vi "Read Analog Input Values.vi"(8 "error in":errorcluster, 9 "Timeout / s":dbl=10.0 format="%0.2f", 10 "AI DAQmx Task":refnum<k21>, 11 "BNT_DAQmx-MCSV in":refnum<class "BNT_DAQmx-MCSV.lvclass">) -> (0 "error out":errorcluster, 1 "AI Data":dbl[](array[numeric]), 3 "BNT_DAQmx-MCSV out":refnum<class "BNT_DAQmx-MCSV.lvclass">)   [LabVIEW 2017, in "BNT_DAQmx.lvlib" / "BNT_DAQmx-MCSV.lvclass"]
doc: "Read analog input.\n\n<b>Default Implementation:</b> Analog Input\n\nThis dynamic dispatch VI can be overritten by derived classes to implement other analog input readings."
uses:
  BNT_DAQmx-MCSV.lvclass
  <vilib>/DAQmx/read.llb/DAQmx Read (Analog 1D DBL NChan 1Samp).vi
  <vilib>/DAQmx/miscellaneous.llb/DAQmx Fill In Error Info.vi
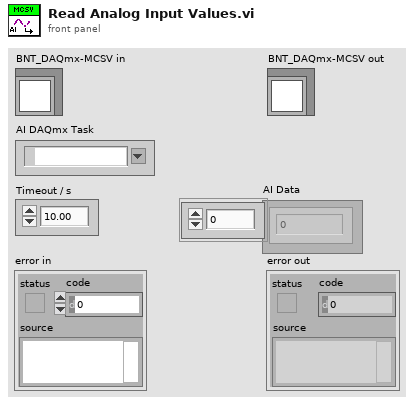
[diagram p1: front panel]
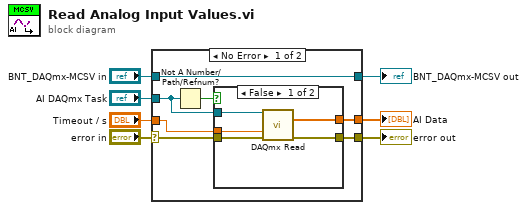
[diagram p0: block diagram]
diagram:
  n1 = case shown="No Error" "error in" {
    selector: "error in" -> [w13 w22]
    tunnel: [w12 w22] -> w6
    tunnel: [w10 w21] -> w4
    tunnel: "BNT_DAQmx-MCSV in" -> [w10 w21]
    tunnel: "Timeout / s" -> [w14 _]
    tunnel: [w11 _] -> w2
    tunnel: "AI DAQmx Task" -> [w8 _]
    frame No Error {
      n2 = Not A Number/Path/Refnum?(number/path/refnum=w8) -> (NaN/Path/Refnum?=w9:bool)
      n3 = case shown="False" w9 {
        tunnel: w14 -> [w19 _]
        tunnel: w13 -> [w18 w20]
        tunnel: [w17 w20] -> w12
        tunnel: [w16 _] -> w11
        tunnel: w8 -> [w15 _]
        frame False {
          n4 = call-poly <vilib>:"DAQmx Read.vi"("task/channels in"=w15, "timeout"=w19, "error in"=w18) -> ("data"=w16:dbl[], "error out"=w17:errorcluster)  [unwired: 10 in, 1 out]
        }
        frame True {
        }
      }
    }
    frame Error {
    }
  }
  "error out" <- w6
  "BNT_DAQmx-MCSV out" <- w4
  "AI Data" <- w2
